vi "write.vi"(8 "error in (no error)":errorcluster, 9 "String":string, 10 "Numeric":dbl, 11 "ValuePass in":refnum<class "RPCVariable.lvclass">) -> (0 "error out":errorcluster, 3 "ValuePass out":refnum<class "RPCVariable.lvclass">)   [LabVIEW 2011, in "mbed_LVLibrary.lvlib" / "RPCVariable.lvclass"]
doc: "This VI writes the RPCVariable on mbed. To write a numeric value connect only the Numeric connection. To write a string (char value) or a number already formatted to a string the connect to the string. When using this VI you need to be aware of the type of the variable this refers to on mbed."
uses:
  RPCVariable.lvclass
  RPCVariable.lvclass/RPCVariable.ctl
  Transport Mechanisms/mbed/mbed.lvclass
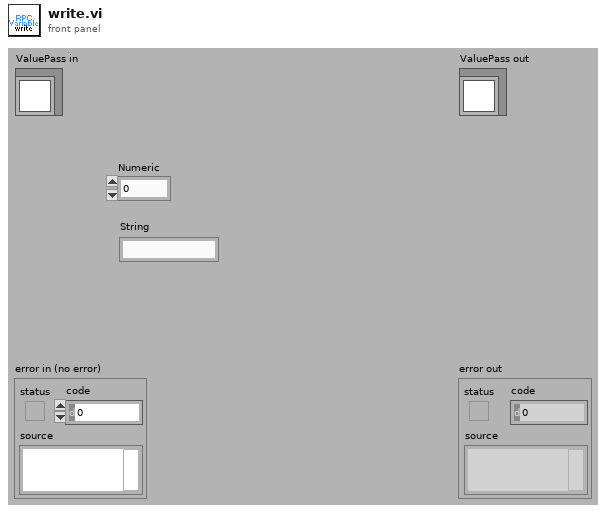
[diagram p1: front panel]
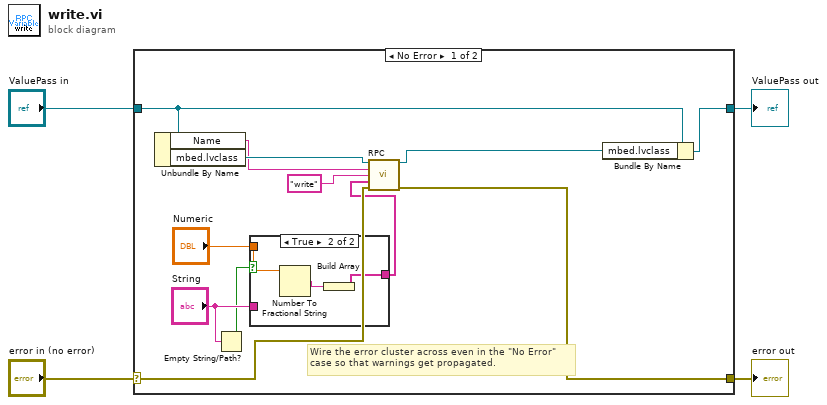
[diagram p0: block diagram]
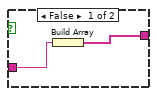
[diagram p2: hidden frame]
diagram:
  n1 = case shown="No Error" "error in (no error)" {
    selector: "error in (no error)" -> [w10 w23]
    tunnel: [w9 w23] -> w3
    tunnel: [w16 w22] -> w1
    tunnel: "ValuePass in" -> [w15 w22]
    frame No Error {
      # "Wire the error cluster across even in the \"No Error\"\ncase so that warnings get propagated."
      n2 = Unbundle By Name(w15) -> ("Name"=w13:string, "mbed.lvclass"=w14:refnum<class "mbed.lvclass">)
      n3 = Empty String/Path?(string/path="String") -> (empty?=w5:bool)
      n4 = case shown="True" w5 {
        tunnel: "Numeric" -> [_ w20]
        tunnel: [w18 w19] -> w8
        tunnel: "String" -> [w17 _]
        frame False {
          n5 = Build Array(w17) -> (w18:string[])
        }
        frame True {
          n6 = Number To Fractional String(number=w20) -> (F-format string=w21:string)  [unwired: 3 in]
          n7 = Build Array(w21) -> (w19:string[])
        }
      }
      n8 = call-dynamic "RPC.vi"("mbed in"=w14, "Name"=w13, "method"="write", "Args"=w8, "error in (no error)"=w10) -> ("mbed out"=w12:refnum<class "mbed.lvclass">, "error out"=w9:errorcluster)  [unwired: 8 in, 1 out]
      n9 = Bundle By Name(cluster=w15, "mbed.lvclass"=w12) -> (w16:refnum<class "RPCVariable.lvclass">)
    }
    frame Error {
    }
  }
  "error out" <- w3
  "ValuePass out" <- w1
